vi "Find optimal B-Spline Parameters.vi"(11 "Input":dbl[](array[numeric])) -> (1 "Residual":dbl, 2 "X":i32[](array[numeric]), 3 "Best BSpline Fit Y":dbl[](array[numeric]))   [LabVIEW 2013, in "main.lvlib"]
uses:
  main.lvlib
  <vilib>/Analysis/NI_AALPro.lvlib
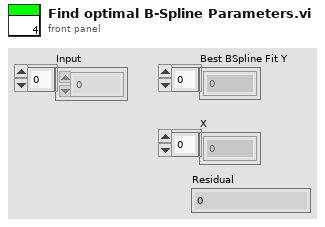
[diagram p1: front panel]
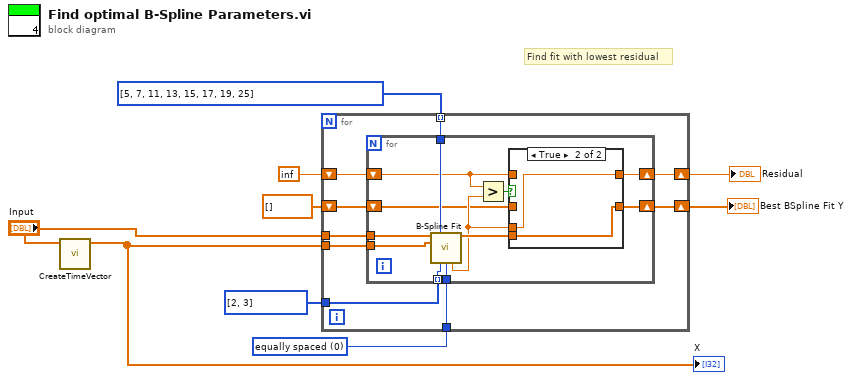
[diagram p0: block diagram]
diagram:
  w9 = u16 0 items=["equally spaced", "chord length", "centripetal"] ("parameter selection")
  # "Find fit with lowest residual"
  n1 = call "CreateTimeVector.vi"("Array in"="Input") -> ("Array out"=w6:dbl[])  [unwired: 10 in]
  "X" <- w6
  n2 = for {
    tunnel: "Input" -> [w11]
    tunnel: w6 -> [w10]
    tunnel: w9 -> [w18]
    tunnel: i32[] [5, 7, 11, 13, 15, 17, 19, 25] -> [w17] mode=indexing
    shift-right: [w13] -> w1
    shift-left: inf -> [w16]
    shift-right: [w14] -> w4
    shift-left: dbl[] [] ("Best BSpline Fit Y") -> [w15]
    tunnel: i32[] [2, 3] -> [w12]
    n3 = for {
      tunnel: w18 -> [w30]
      tunnel: w17 -> [w29]
      tunnel: w12 -> [w21] mode=indexing
      tunnel: w11 -> [w20]
      tunnel: w10 -> [w19]
      shift-right: [w22] -> w13
      shift-left: w16 -> [w25]
      shift-right: [w23] -> w14
      shift-left: w15 -> [w24]
      n4 = call <vilib>:"B-Spline Fit.vi"("Y"=w20, "# of control points"=w29, "X"=w19, "degree"=w21, "parameter selection"=w30) -> ("Best BSpline Fit Y"=w27:dbl[], "residue"=w26:dbl)  [unwired: 7 in, 2 out]
      n5 = Greater?(x=w25, y=w26) -> (0:w28:bool)
      n6 = case shown="True" w28 {
        tunnel: w26 -> [_ w34]
        tunnel: [w32 w34] -> w22
        tunnel: w25 -> [w32 _]
        tunnel: w27 -> [_ w33]
        tunnel: [w31 w33] -> w23
        tunnel: w24 -> [w31 _]
        frame False {
        }
        frame True {
        }
      }
    }
  }
  "Best BSpline Fit Y" <- w4
  "Residual" <- w1
